vi "Package Calibration Results.vi"(6 "Filter Sequences":T2[](array[typedef]), 8 "error in (no error)":errorcluster, 11 "calResult":refnum<k24>) -> (0 "error out":errorcluster, 3 "Filter Results":T1[](array[typedef]))   [LabVIEW 2015]
uses:
  Controls/Filter Sequence.ctl
  Controls/Filter Result.ctl
  C:/Distributed/CalFlex.dll
  CalFlex.dll
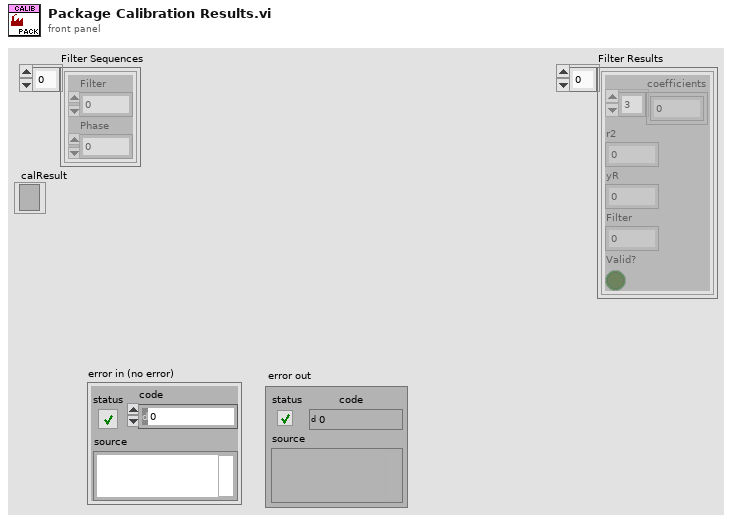
[diagram p1: front panel]
types:
  T1 = typedef "Filter Result.ctl" = cluster{"coefficients":dbl[], "r2":dbl, "yR":dbl, "Filter":i32, "Valid?":bool}
  T2 = typedef "Filter Sequence.ctl" = cluster{"Filter":u8, "Phase":dbl}
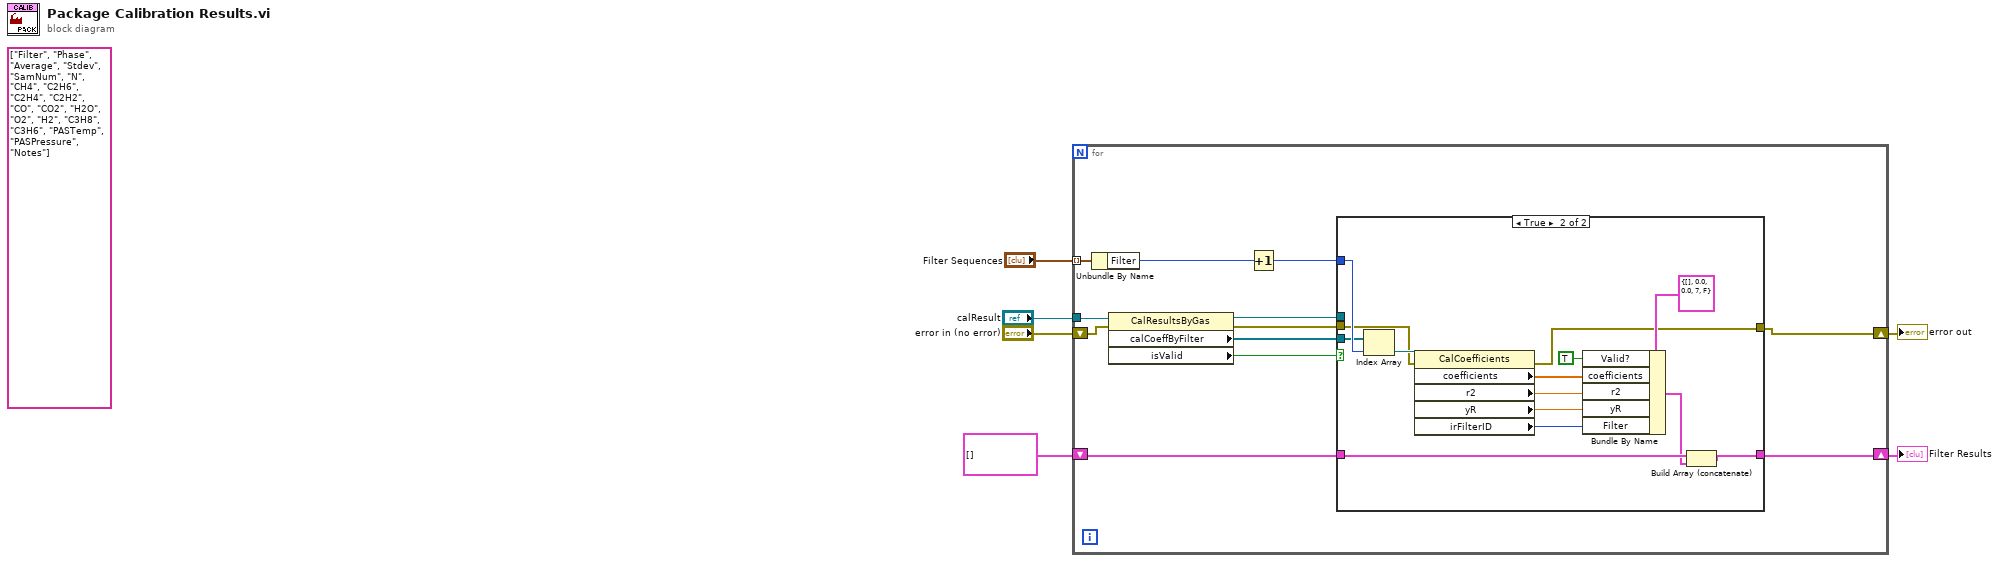
[diagram p0: block diagram]
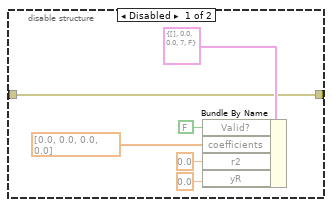
[diagram p3: hidden frame]
diagram:
  (unwired) string[] ["Filter", "Phase", "Average", "Stdev", "SamNum", "N", "CH4", "C2H6", "C2H4", "C2H2", "CO", "CO2", "H2O", "O2", "H2", "C3H8", "C3H6", "PASTemp", "PASPressure", "Notes"]
  n1 = for {
    tunnel: "Filter Sequences" -> [w18] mode=indexing
    tunnel: "calResult" -> [w17]
    shift-right: [w9] -> w3
    shift-left: T1[] [] -> [w10]
    shift-right: [w8] -> w2
    shift-left: "error in (no error)" -> [w16]
    n2 = Unbundle By Name(w18) -> ("Filter"=w11:u8)
    n3 = property class="CalResultsByGas"(reference=w17, error in=w16) -> (reference out=w12:refnum<k24>, error out=w13:errorcluster, "calCoeffByFilter"=w14:refnum<k24>[], "isValid"=w15:bool)
    n4 = Increment(x=w11) -> (x+1=w7:u8)
    n5 = case shown="True" w15 {
      tunnel: w14 -> [_ w41]
      tunnel: w7 -> [_ w42]
      tunnel: w13 -> [w20 w38]
      tunnel: w12 -> [_ _]
      tunnel: [w21 w31] -> w9
      tunnel: w10 -> [w21 w33]
      tunnel: [w19 w30] -> w8
      frame False {
        n6 = disable-structure shown="Enabled" {
          disable-tunnel: w20 -> [w22 w28]
          disable-tunnel: [w22 w28] -> w19
          frame Disabled {
            n7 = Bundle By Name(cluster=T1 {"coefficients"=[], "r2"=0.0, "yR"=0.0, "Filter"=7, "Valid?"=FALSE} ("Filter Result"), "Valid?"=FALSE, "coefficients"=dbl[] [0.0, 0.0, 0.0, 0.0], "r2"=0.0, "yR"=0.0) -> ()  [unwired: 1 out]
          }
          frame Enabled {
          }
        }
      }
      frame True {
        n8 = Index Array(array=w41, index=w42) -> (element=w39:refnum<k24>)
        n9 = property class="CalCoefficients"(reference=w39, error in=w38) -> (error out=w30:errorcluster, "coefficients"=w37:dbl[], "r2"=w36:dbl, "yR"=w35:dbl, "irFilterID"=w29:i32)  [unwired: 1 out]
        n10 = Bundle By Name(cluster=T1 {"coefficients"=[], "r2"=0.0, "yR"=0.0, "Filter"=7, "Valid?"=FALSE} ("Filter Result"), "Valid?"=TRUE, "coefficients"=w37, "r2"=w36, "yR"=w35, "Filter"=w29) -> (w32:T1)
        n11 = Build Array (concatenate)(w33, w32) -> (w31:T1[])
      }
    }
  }
  "Filter Results" <- w3
  "error out" <- w2
